vi "Get Keithley Data.vi"(6 "GPIB = true, RS-232 = false":bool, 7 "wait after write (ms)":u32, 8 "error in (no error)":errorcluster, 10 "Command":string, 11 "VISA resource name":refnum<visa-resource-name>) -> (0 "error out":errorcluster, 1 "Data String":string, 2 "Data":dbl[](array[numeric]), 3 "VISA resource name out":refnum<visa-resource-name>)   [LabVIEW 2018]
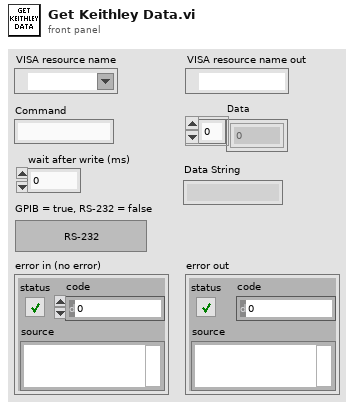
[diagram p1: front panel]
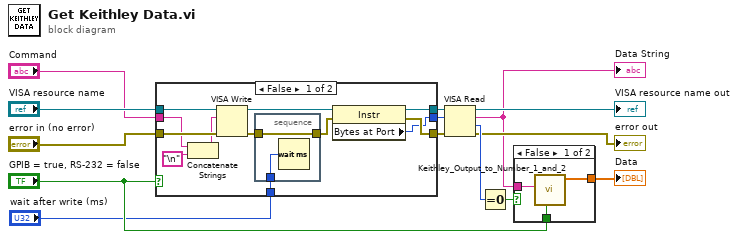
[diagram p0: block diagram]
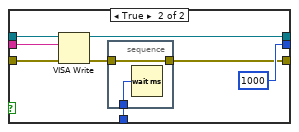
[diagram p2: hidden frame]
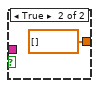
[diagram p3: hidden frame]
diagram:
  n1 = case shown="False" "GPIB = true, RS-232 = false" {
    tunnel: "VISA resource name" -> [w19 w31]
    tunnel: "error in (no error)" -> [w21 w33]
    tunnel: [w23 u32 1000 ("byte count")] -> w9
    tunnel: [w26 w30] -> w8
    tunnel: [w24 w35] -> w7
    tunnel: "wait after write (ms)" -> [w22 w34]
    tunnel: "Command" -> [w15 w29]
    frame False {
      n2 = Concatenate Strings(w15, "\n") -> (w16:string)
      n3 = VISA Write(VISA resource name=w19, write buffer=w16, error in (no error)=w21) -> (VISA resource name out=w18:refnum<visa-resource-name>, error out=w20:errorcluster)  [unwired: 1 out]
      n4 = stacked-sequence {
        tunnel: w20 -> [w28]
        tunnel: [w28] -> w25
        tunnel: w22 -> [w27]
        frame #0 {
          n5 = Wait (ms)(milliseconds to wait=w27) -> ()  [unwired: 1 out]
        }
      }
      n6 = property class="Instr"(reference=w18, error in=w25) -> (reference out=w26:refnum<visa-resource-name>, error out=w24:errorcluster, "Bytes at Port"=w23:u32)
    }
    frame True {
      n7 = VISA Write(VISA resource name=w31, write buffer=w29, error in (no error)=w33) -> (VISA resource name out=w30:refnum<visa-resource-name>, error out=w32:errorcluster)  [unwired: 1 out]
      n8 = stacked-sequence {
        tunnel: w32 -> [w38]
        tunnel: [w38] -> w35
        tunnel: w34 -> [w37]
        frame #0 {
          n9 = Wait (ms)(milliseconds to wait=w37) -> ()  [unwired: 1 out]
        }
      }
    }
  }
  n10 = VISA Read(VISA resource name=w8, byte count=w9, error in (no error)=w7) -> (VISA resource name out=→"VISA resource name out":refnum<visa-resource-name>, read buffer=w4:string, return count=w14:u32, error out=→"error out":errorcluster)
  "Data String" <- w4
  n11 = Equal To 0?(x=w14) -> (x = 0?=w13:bool)
  n12 = case shown="False" w13 {
    tunnel: [w41 dbl[] [] ("array")] -> w10
    tunnel: w4 -> [w40 _]
    tunnel: "GPIB = true, RS-232 = false" -> [w39 _]
    frame False {
      n13 = call "Keithley_Output_to_Number_1_and_2.vi"("GPIB = true, RS-232 = false"=w39, "string"=w40) -> ("array"=w41:dbl[])  [unwired: 7 in, 2 out]
    }
    frame True {
    }
  }
  "Data" <- w10
